vi "OnStopMotion.vi"(8 "error in":errorcluster, 9 "In Motion":refnum<vi>, 10 "Go":refnum<vi>, 11 "CmdLib In":refnum<k24>) -> (0 "error out":errorcluster)   [LabVIEW 2009]
uses:
  C:/Code/Apps/Utilities/Picomotor/PicomotorApp/Install/Samples/LabVIEW/Model 8743/LabVIEW 2009/CmdLib.dll
  Global Variables.vi
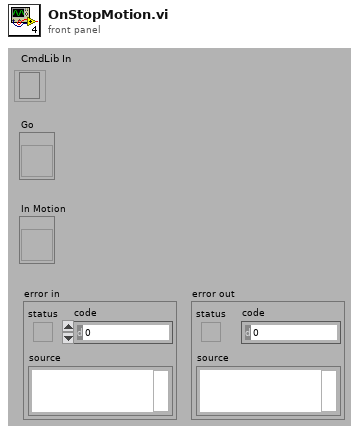
[diagram p1: front panel]
types:
  T1 = enum8{"Enabled", "Disabled", "Disabled and Grayed Out"}
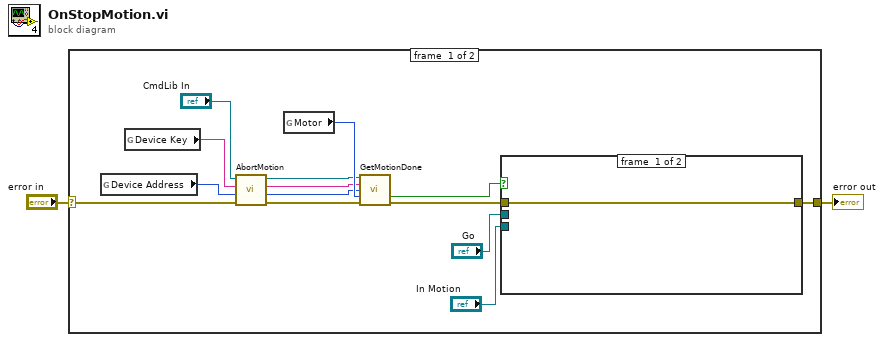
[diagram p0: block diagram]
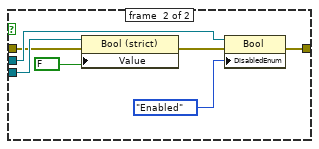
[diagram p2: hidden frame]
diagram:
  n1 = case shown="No Error" "error in" {
    selector: "error in" -> [w4 w25]
    tunnel: [w13 w25] -> w2
    frame #0 {
      n2 = global read "Global Variables.vi" "Device Address"() -> (w7:i32)
      n3 = global read "Global Variables.vi" "Device Key"() -> (w6:string)
      n4 = call "AbortMotion.vi"("error in (no error)"=w4, "Device Address In"=w7, "DeviceKey In"=w6, "CmdLib In"="CmdLib In") -> ("error out"=w8:errorcluster, "Device Address Out"=w11:i32, "DeviceKey Out"=w10:string, "CmdLib Out"=w9:refnum<k24>)
      n5 = global read "Global Variables.vi" "Motor"() -> (w12:i32)
      n6 = call "GetMotionDone.vi"("CmdLib In"=w9, "DeviceKey In"=w10, "Device Address In"=w11, "Motor"=w12, "error in (no error)"=w8) -> ("Is Motion Done"=w15:bool, "error out"=w14:errorcluster)  [unwired: 6 in, 3 out]
      n7 = case shown="True" w15 {
        tunnel: [w17 w18] -> w13
        tunnel: "Go" -> [_ w23]
        tunnel: w14 -> [w17 w20]
        tunnel: "In Motion" -> [_ w22]
        frame #0 {
        }
        frame #1 {
          n8 = property class="Bool (strict)"(reference=w22, error in=w20, "Value"=FALSE) -> (error out=w19:errorcluster)  [unwired: 1 out]
          n9 = property class="Bool"(reference=w23, error in=w19, "DisabledEnum"=T1."Enabled" ("Disabled")) -> (error out=w18:errorcluster)  [unwired: 1 out]
        }
      }
    }
    frame #1 {
    }
  }
  "error out" <- w2
